vi "Tree.Update.vi"(5 "Group Channels?":bool, 7 "Report Passed?":bool, 8 "error in (no error)":errorcluster, 9 "Results":variant, 10 "TreeControl in":refnum<vi>, 11 "Data Path":path) -> (0 "error out":errorcluster, 1 "Passed?":bool, 2 "Tree Ref":refnum<vi>, 3 "Data Path":path)   [LabVIEW 2015, in "NIAnalysis.lvlib"]
uses:
  NIAnalysis.lvlib
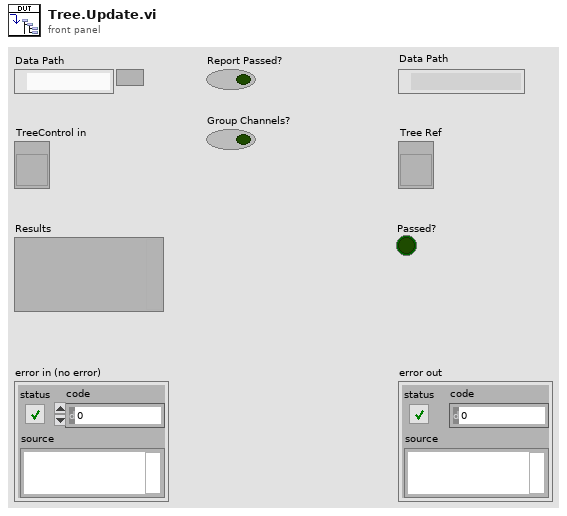
[diagram p1: front panel]
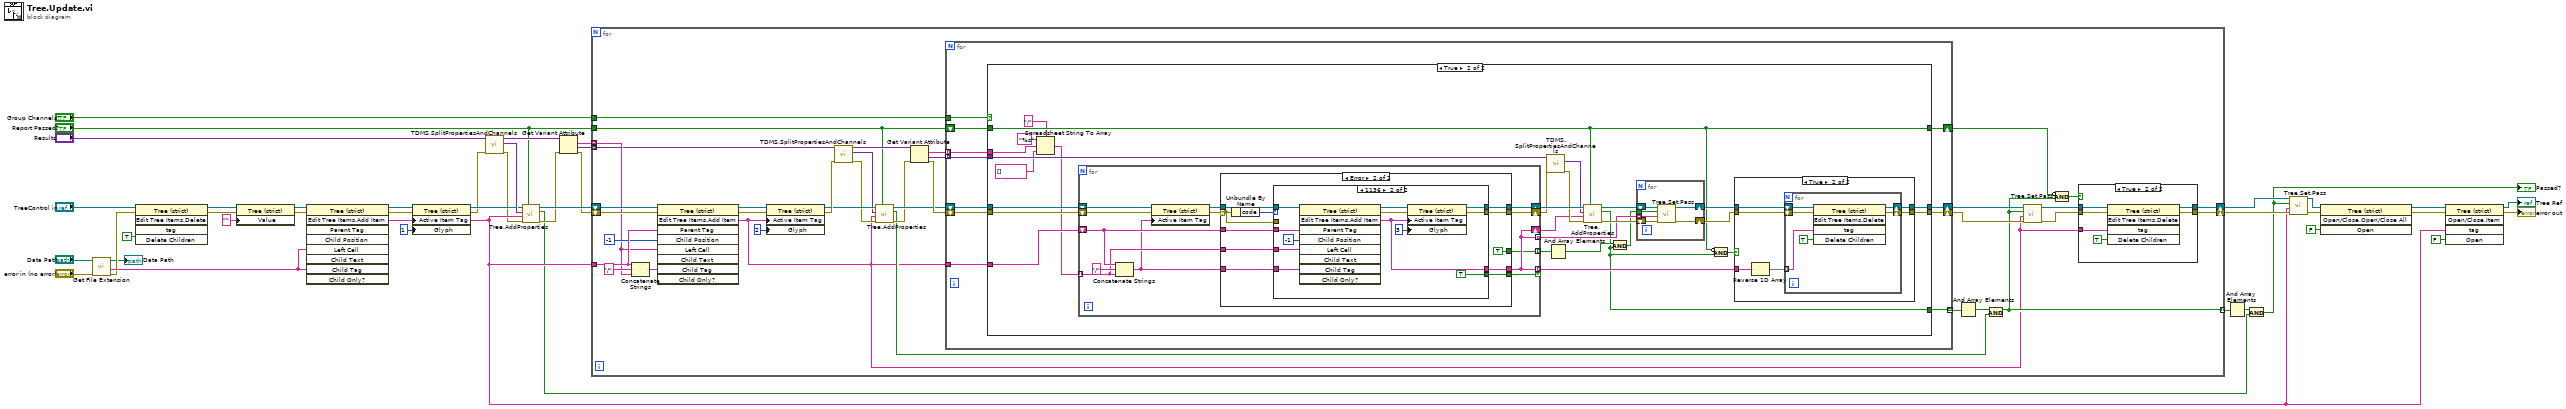
[diagram p0: block diagram]
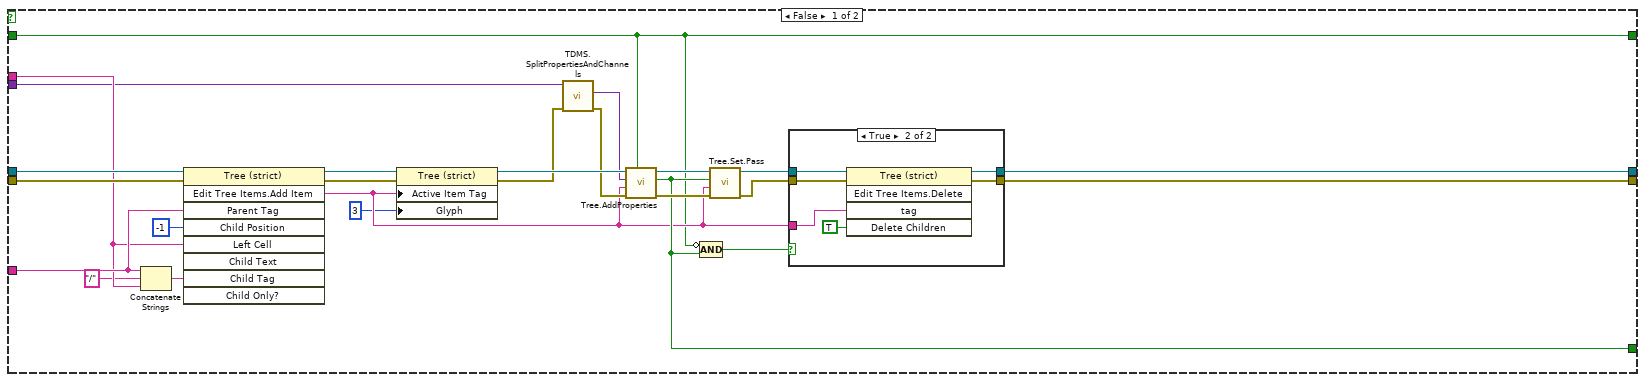
[diagram p2: hidden frame]
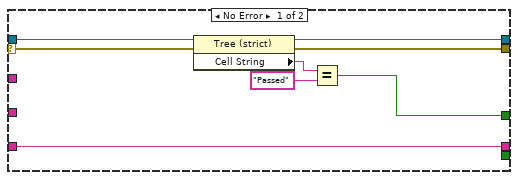
[diagram p4: hidden frame]
diagram:
  n1 = call <vilib>:"Get File Extension.vi"("error in (no error)"="error in (no error)", "file"="Data Path") -> ("error out"=w6:errorcluster, "filename without extension"=w35:string, "dup file"=→"Data Path":path)  [unwired: 5 in, 2 out]
  n2 = invoke class="Tree (strict)" method="Edit Tree Items.Delete"(reference="TreeControl in", error in=w6, "Delete Children"=TRUE ("Delete Children?")) -> (reference out=w26:refnum<vi>, error out=w25:errorcluster)  [unwired: 2 in, 3 out]
  n3 = property class="Tree (strict)"(reference=w26, error in=w25, "Value"="" ("Active Item:Tag")) -> (reference out=w23:refnum<vi>, error out=w24:errorcluster)
  n4 = invoke class="Tree (strict)" method="Edit Tree Items.Add Item"(reference=w23, error in=w24, "Left Cell"=w35, "Child Tag"=w35) -> (reference out=w33:refnum<vi>, error out=w32:errorcluster, "Edit Tree Items:Add Item"=w17:string)  [unwired: 5 in, 6 out]
  n5 = property class="Tree (strict)"(reference=w33, error in=w32, "Active Item Tag"=w17, "Glyph"=1 ("Active Item:Symbol Index")) -> (reference out=w19:refnum<vi>, error out=w5:errorcluster)
  n6 = call "TDMS.SplitPropertiesAndChannels.vi"("error in"=w5, "Properties"="Results") -> ("error out"=w4:errorcluster, "Properties"=w20:variant, "Channels"=w16:variant)  [unwired: 7 in]
  n7 = call "Tree.AddProperties.vi"("Report Passed?"="Report Passed?", "error in (no error)"=w4, "Parent"=w17, "Properties"=w20, "Tree Ref"=w19) -> ("error out"=w15:errorcluster, "Passed?"=w9:bool, "Tree Ref"=w18:refnum<vi>)  [unwired: 4 in]
  n8 = Get Variant Attribute(Variant=w16, error in=w15) -> (names=w13:string[], values=w12:variant[], error out=w14:errorcluster)  [unwired: 2 in, 1 out]
  n9 = for {
    tunnel: w13 -> [w63] mode=indexing
    tunnel: w12 -> [w62] mode=indexing
    shift-right: [w49] -> w40
    shift-left: w14 -> [w78]
    tunnel: [w51] -> w41 mode=indexing
    tunnel: w17 -> [w70]
    shift-right: [w47] -> w39
    shift-left: w18 -> [w79]
    tunnel: "Report Passed?" -> [w53]
    tunnel: "Group Channels?" -> [w44]
    n10 = Concatenate Strings(w70, "/" ("string"), w63) -> (w71:string)
    n11 = invoke class="Tree (strict)" method="Edit Tree Items.Add Item"(reference=w79, error in=w78, "Parent Tag"=w70, "Child Position"=-1, "Left Cell"=w63, "Child Tag"=w71) -> (reference out=w77:refnum<vi>, error out=w76:errorcluster, "Edit Tree Items:Add Item"=w46:string)  [unwired: 3 in, 6 out]
    n12 = property class="Tree (strict)"(reference=w77, error in=w76, "Active Item Tag"=w46, "Glyph"=2 ("Active Item:Symbol Index")) -> (reference out=w59:refnum<vi>, error out=w60:errorcluster)
    n13 = call "TDMS.SplitPropertiesAndChannels.vi"("error in"=w60, "Properties"=w62) -> ("error out"=w57:errorcluster, "Properties"=w55:variant, "Channels"=w61:variant)  [unwired: 7 in]
    n14 = call "Tree.AddProperties.vi"("Report Passed?"=w53, "error in (no error)"=w57, "Parent"=w46, "Properties"=w55, "Tree Ref"=w59) -> ("error out"=w56:errorcluster, "Passed?"=w54:bool, "Tree Ref"=w58:refnum<vi>)  [unwired: 4 in]
    n15 = Get Variant Attribute(Variant=w61, error in=w56) -> (names=w69:string[], values=w67:variant[], error out=w68:errorcluster)  [unwired: 2 in, 1 out]
    n16 = for {
      tunnel: w69 -> [w87] mode=indexing
      shift-right: [w85] -> w75
      shift-left: w68 -> [w89]
      tunnel: w46 -> [w88]
      tunnel: w67 -> [w82] mode=indexing
      shift-right: [w84] -> w74
      shift-left: w58 -> [w90]
      tunnel: [w86] -> w66 mode=indexing
      shift-right: [w81] -> w45
      shift-left: w53 -> [w83]
      tunnel: w44 -> [w80]
      n17 = case shown="True" w80 {
        tunnel: w90 -> [w115 w151]
        tunnel: w89 -> [w114 w150]
        tunnel: w88 -> [w113 w149]
        tunnel: w87 -> [w106 w135]
        tunnel: [w105 w125] -> w86
        tunnel: [w103 w141] -> w85
        tunnel: [w101 w139] -> w84
        tunnel: w83 -> [w91 w136]
        tunnel: w82 -> [w98 w137]
        tunnel: [w91 w136] -> w81
        frame False {
          n18 = Concatenate Strings(w113, "/" ("string"), w106) -> (w96:string)
          n19 = invoke class="Tree (strict)" method="Edit Tree Items.Add Item"(reference=w115, error in=w114, "Parent Tag"=w113, "Child Position"=-1, "Left Cell"=w106, "Child Tag"=w96) -> (reference out=w95:refnum<vi>, error out=w94:errorcluster, "Edit Tree Items:Add Item"=w100:string)  [unwired: 3 in, 6 out]
          n20 = property class="Tree (strict)"(reference=w95, error in=w94, "Active Item Tag"=w100, "Glyph"=3 ("Active Item:Symbol Index")) -> (reference out=w110:refnum<vi>, error out=w108:errorcluster)
          n21 = call "TDMS.SplitPropertiesAndChannels.vi"("error in"=w108, "Properties"=w98) -> ("error out"=w109:errorcluster, "Properties"=w107:variant)  [unwired: 7 in, 1 out]
          n22 = call "Tree.AddProperties.vi"("Report Passed?"=w91, "error in (no error)"=w109, "Parent"=w100, "Properties"=w107, "Tree Ref"=w110) -> ("error out"=w112:errorcluster, "Passed?"=w105:bool, "Tree Ref"=w111:refnum<vi>)  [unwired: 4 in]
          n23 = Compound Arithmetic op=AND(invert w91, w105) -> (w99:bool)
          n24 = call "Tree.Set.Pass.vi"("error in (no error)"=w112, "Edit Tree Items:Add Item"=w100, "Passed"=w105, "TreeControl in"=w111) -> ("error out"=w104:errorcluster, "TreeControl out"=w102:refnum<vi>)  [unwired: 6 in]
          n25 = case shown="True" w99 {
            tunnel: w104 -> [w117 w122]
            tunnel: [w117 w121] -> w103
            tunnel: w102 -> [w116 w120]
            tunnel: [w116 w119] -> w101
            tunnel: w100 -> [_ w118]
            frame False {
            }
            frame True {
              n26 = invoke class="Tree (strict)" method="Edit Tree Items.Delete"(reference=w120, error in=w122, "tag"=w118, "Delete Children"=TRUE ("Delete Children?")) -> (reference out=w119:refnum<vi>, error out=w121:errorcluster)  [unwired: 1 in, 3 out]
            }
          }
        }
        frame True {
          n27 = Spreadsheet String To Array(delimiter (Tab)="/", format string="%s", spreadsheet string=w135, array type (2D Dbl)=string[] []) -> (array=w130:string[])
          n28 = for {
            tunnel: w130 -> [w166] mode=indexing
            shift-right: [w169] -> w146
            shift-left: w151 -> [w164]
            shift-right: [w168] -> w144
            shift-left: w150 -> [w163]
            shift-right: [w159] -> w131
            shift-left: w149 -> [w170]
            tunnel: [w159] -> w129 mode=indexing if=w160
            tunnel: [w159] -> w128 mode=indexing
            tunnel: [w158] -> w127 mode=indexing
            n29 = Concatenate Strings(w170, "/" ("string"), w166) -> (w165:string)
            n30 = property class="Tree (strict)"(reference=w164, error in=w163, "Active Item Tag"=w165) -> (reference out=w162:refnum<vi>, error out=w161:errorcluster)
            n31 = case shown="Error" w161 {
              selector: w161 -> [w177 w181]
              tunnel: w170 -> [_ w189]
              tunnel: [w174 w188] -> w169
              tunnel: [w176 w187] -> w168
              tunnel: w166 -> [_ w186]
              tunnel: [w178 w185] -> w159
              tunnel: w165 -> [w178 w184]
              tunnel: w162 -> [w175 w183]
              tunnel: [_ w180] -> w160
              tunnel: [w171 TRUE] -> w158
              frame No Error {
                n32 = property class="Tree (strict)"(reference=w175, error in=w177) -> (reference out=w174:refnum<vi>, error out=w176:errorcluster, "Cell String"=w172:string)
                n33 = Equal?(x=w172, y="Passed") -> (x = y?=w171:bool)
              }
              frame Error {
                n34 = Unbundle By Name(w181) -> ("code"=w182:i32)
                n35 = case shown="1136" w182 {
                  tunnel: w189 -> [_ w204]
                  tunnel: [w192 w203] -> w188
                  tunnel: [w191 w202] -> w187
                  tunnel: w186 -> [_ w199]
                  tunnel: [w190 w197] -> w185
                  tunnel: w184 -> [w190 w196]
                  tunnel: w183 -> [w192 w195]
                  tunnel: w181 -> [w191 _]
                  tunnel: [_ TRUE] -> w180
                  frame Default {
                  }
                  frame 1136 {
                    n36 = invoke class="Tree (strict)" method="Edit Tree Items.Add Item"(reference=w195, "Parent Tag"=w204, "Child Position"=-1, "Left Cell"=w199, "Child Tag"=w196) -> (reference out=w198:refnum<vi>, error out=w201:errorcluster, "Edit Tree Items:Add Item"=w197:string)  [unwired: 4 in, 6 out]
                    n37 = property class="Tree (strict)"(reference=w198, error in=w201, "Active Item Tag"=w197, "Glyph"=3 ("Active Item:Symbol Index")) -> (reference out=w203:refnum<vi>, error out=w202:errorcluster)
                  }
                }
              }
            }
          }
          n38 = call "TDMS.SplitPropertiesAndChannels.vi"("error in"=w144, "Properties"=w137) -> ("error out"=w145:errorcluster, "Properties"=w143:variant)  [unwired: 7 in, 1 out]
          n39 = And Array Elements(Boolean array=w127) -> (logical AND=w126:bool)
          n40 = call "Tree.AddProperties.vi"("Report Passed?"=w136, "error in (no error)"=w145, "Parent"=w131, "Properties"=w143, "Tree Ref"=w146) -> ("error out"=w148:errorcluster, "Passed?"=w125:bool, "Tree Ref"=w147:refnum<vi>)  [unwired: 4 in]
          n41 = Compound Arithmetic op=AND(w126, w125) -> (w124:bool)
          n42 = for {
            tunnel: w124 -> [w155]
            tunnel: w128 -> [w152] mode=indexing
            shift-right: [w154] -> w142
            shift-left: w148 -> [w157]
            shift-right: [w153] -> w140
            shift-left: w147 -> [w156]
            n43 = call "Tree.Set.Pass.vi"("error in (no error)"=w157, "Edit Tree Items:Add Item"=w152, "Passed"=w155, "TreeControl in"=w156) -> ("error out"=w154:errorcluster, "TreeControl out"=w153:refnum<vi>)  [unwired: 6 in]
          }
          n44 = Compound Arithmetic op=AND(invert w136, w125) -> (w138:bool)
          n45 = case shown="True" w138 {
            tunnel: w142 -> [w206 w212]
            tunnel: [w206 w211] -> w141
            tunnel: w140 -> [w205 w210]
            tunnel: [w205 w209] -> w139
            tunnel: w129 -> [_ w208]
            frame False {
            }
            frame True {
              n46 = Reverse 1D Array(array=w208) -> (reversed array=w207:string[])
              n47 = for {
                tunnel: w207 -> [w213] mode=indexing
                shift-right: [w216] -> w211
                shift-left: w212 -> [w217]
                shift-right: [w214] -> w209
                shift-left: w210 -> [w215]
                n48 = invoke class="Tree (strict)" method="Edit Tree Items.Delete"(reference=w215, error in=w217, "tag"=w213, "Delete Children"=TRUE ("Delete Children?")) -> (reference out=w214:refnum<vi>, error out=w216:errorcluster)  [unwired: 1 in, 3 out]
              }
            }
          }
        }
      }
    }
    n49 = And Array Elements(Boolean array=w66) -> (logical AND=w73:bool)
    n50 = Compound Arithmetic op=AND(w73, w54) -> (w51:bool)
    n51 = call "Tree.Set.Pass.vi"("error in (no error)"=w75, "Edit Tree Items:Add Item"=w46, "Passed"=w51, "TreeControl in"=w74) -> ("error out"=w50:errorcluster, "TreeControl out"=w48:refnum<vi>)  [unwired: 6 in]
    n52 = Compound Arithmetic op=AND(invert w45, w51) -> (w52:bool)
    n53 = case shown="True" w52 {
      tunnel: w50 -> [w220 w225]
      tunnel: [w220 w224] -> w49
      tunnel: w48 -> [w219 w223]
      tunnel: [w219 w222] -> w47
      tunnel: w46 -> [_ w221]
      frame False {
      }
      frame True {
        n54 = invoke class="Tree (strict)" method="Edit Tree Items.Delete"(reference=w223, error in=w225, "tag"=w221, "Delete Children"=TRUE ("Delete Children?")) -> (reference out=w222:refnum<vi>, error out=w224:errorcluster)  [unwired: 1 in, 3 out]
      }
    }
  }
  n55 = And Array Elements(Boolean array=w41) -> (logical AND=w11:bool)
  n56 = Compound Arithmetic op=AND(w11, w9) -> (w10:bool)
  "Passed?" <- w10
  n57 = call "Tree.Set.Pass.vi"("error in (no error)"=w40, "Edit Tree Items:Add Item"=w17, "Passed"=w10, "TreeControl in"=w39) -> ("error out"=w36:errorcluster, "TreeControl out"=w37:refnum<vi>)  [unwired: 6 in]
  n58 = invoke class="Tree (strict)" method="Open/Close.Open/Close All"(reference=w37, error in=w36, "Open"=FALSE ("Open?")) -> (reference out=w30:refnum<vi>, error out=w29:errorcluster)  [unwired: 1 in, 2 out]
  n59 = invoke class="Tree (strict)" method="Open/Close.Item"(reference=w30, error in=w29, "tag"=w17, "Open"=FALSE ("Open?")) -> (reference out=→"Tree Ref":refnum<vi>, error out=→"error out":errorcluster)  [unwired: 1 in, 3 out]
